vi "niFPGA I32xU16 - MSB.vi"(2 "A":i32, 3 "B":u16) -> (7 "A*B [Hi I32]":i32=2838 format="%08x")   [LabVIEW 2017]
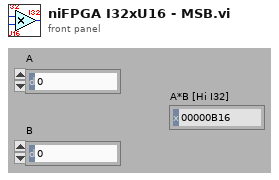
[diagram p1: front panel]
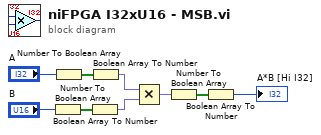
[diagram p0: block diagram]
diagram:
  n1 = Number To Boolean Array(number="B") -> (Boolean array=w7:bool[])
  n2 = Number To Boolean Array(number="A") -> (Boolean array=w9:bool[])
  n3 = Boolean Array To Number(Boolean array=w7) -> (number=w5:fxp<+,16,0>)
  n4 = Boolean Array To Number(Boolean array=w9) -> (number=w4:fxp<+/-,32,0>)
  n5 = Multiply(x=w4, y=w5) -> (x*y=w2:fxp<+/-,32,0>)
  n6 = Number To Boolean Array(number=w2) -> (Boolean array=w3:bool[])
  n7 = Boolean Array To Number(Boolean array=w3) -> (number=→"A*B [Hi I32]":i32)
